vi "subReadIncrementalBuildInfoFromFile.vi"(8 "error in (no error)":errorcluster, 11 "SolutionBuilder in":refnum<class "SolutionBuilder.lvclass">) -> (0 "error out":errorcluster, 3 "SolutionBuilder out":refnum<class "SolutionBuilder.lvclass">)   [LabVIEW 2019, in "SolutionBuilder.lvlib" / "SolutionBuilder.lvclass"]
uses:
  SolutionBuilder.lvclass
  <vilib>/Utility/config.llb/NI_LVConfig.lvlib
  BuildManager/BuildProjectInfo.ctl
  BuildManager/BuildManager.lvclass
  IncrementalFileInfoHash.ctl
  <vilib>/Utility/miscctls.llb/LVMapReplaceAction.ctl
  <vilib>/Utility/config.llb/Read Key (String).vi
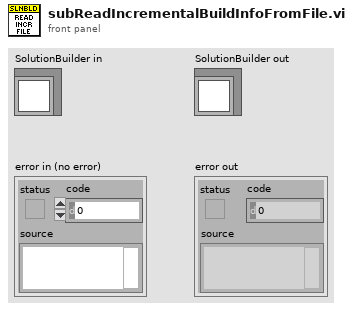
[diagram p1: front panel]
types:
  T1 = typedef "SolutionBuilder.lvlib/BuildManager.lvclass/BuildProjectInfo.ctl" = cluster{"Project path":string, "Build spec name":string, "Target":string}
  T2 = typedef "SolutionBuilder.lvlib/SolutionBuilder.lvclass/IncrementalFileInfoHash.ctl" = cluster{"Project path":string, "Build spec name":string, "Target":string, "File":string, "MD5 hash":string}
  T3 = typedef "LVMapReplaceAction.ctl" = enum32{"Modify Entry only if found", "Add or Modify Entry", "Delete Entry"}
  T4 = typedef "NI_LVConfig.lvlib/Config Data RefNum.ctl" = refnum<k1>
  T5 = typedef "SolutionBuilder.lvlib/SolutionBuilder.lvclass/HashMap.ctl" = map{T1, map{string, string}}
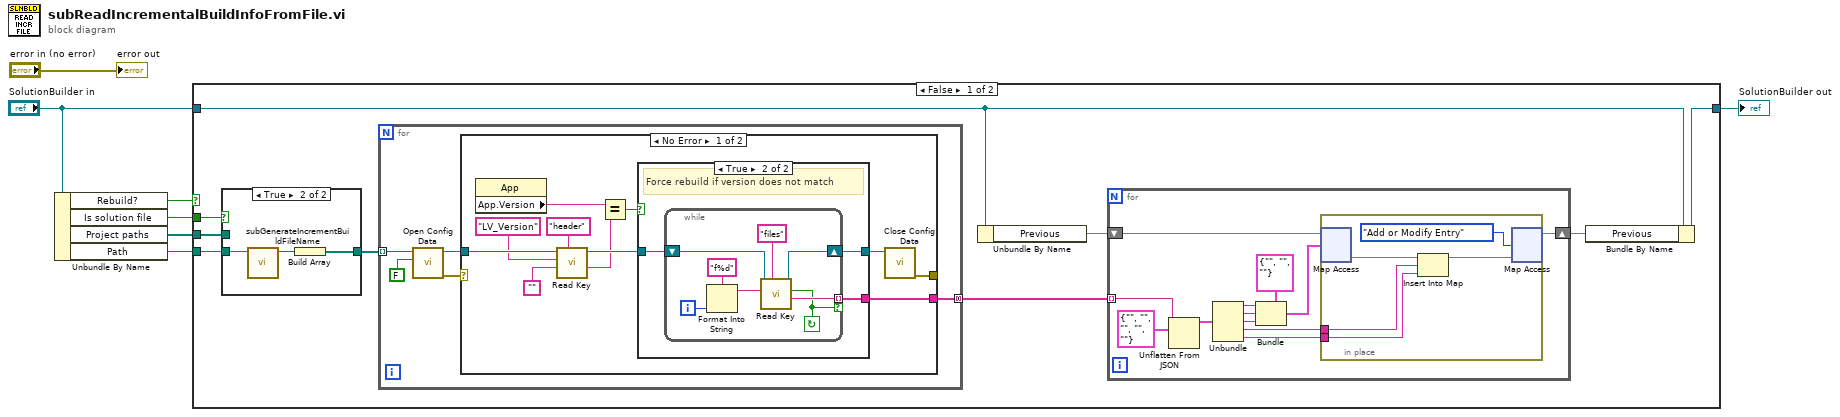
[diagram p0: block diagram]
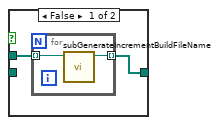
[diagram p4: hidden frame]
diagram:
  n1 = Unbundle By Name("SolutionBuilder in") -> ("Rebuild?"=w1:bool, "Is solution file"=w6:bool, "Project paths"=w4:path[], "Path"=w5:path)
  n2 = case shown="False" w1 {
    tunnel: w6 -> [w16 _]
    tunnel: w5 -> [w15 _]
    tunnel: w4 -> [w14 _]
    tunnel: [w10 w69] -> w3
    tunnel: "SolutionBuilder in" -> [w9 w69]
    frame False {
      n3 = case shown="True" w16 {
        tunnel: w15 -> [_ w51]
        tunnel: w14 -> [w46 _]
        tunnel: [w45 w49] -> w13
        frame False {
          n4 = for {
            tunnel: w46 -> [w48] mode=indexing
            tunnel: [w47] -> w45 mode=indexing
            n5 = call "subGenerateIncrementBuildFileName.vi"("Path in"=w48) -> ("Path out"=w47:path)  [unwired: 10 in]
          }
        }
        frame True {
          n6 = call "subGenerateIncrementBuildFileName.vi"("Path in"=w51) -> ("Path out"=w50:path)  [unwired: 10 in]
          n7 = Build Array(w50) -> (w49:path[])
        }
      }
      n8 = for {
        tunnel: w13 -> [w19] mode=indexing
        tunnel: [w18] -> w12 mode=concatenating
        n9 = call <vilib>:"Open Config Data.vi"("create file if necessary (T)"=FALSE, "configuration file path"=w19) -> ("error out"=w20:errorcluster, "refnum"=w21:T4)  [unwired: 7 in, 1 out]
        n10 = case shown="No Error" w20 {
          tunnel: w21 -> [w29 _]
          tunnel: [w31 _] -> _
          tunnel: [w30 _] -> w18
          frame No Error {
            n11 = property class="App"() -> ("App.Version"=w24:string)  [unwired: 2 in, 2 out]
            n12 = call-poly <vilib>:"Read Key.vi"("section"="header", "default value"="", "key"="LV_Version", "refnum"=w29) -> ("value"=w22:string, "refnum out"=w28:T4)  [unwired: 4 in, 2 out]
            n13 = Equal?(x=w24, y=w22) -> (x = y?=w23:bool)
            n14 = case shown="True" w23 {
              tunnel: [w33 w36] -> w32
              tunnel: [_ w35] -> w30
              tunnel: w28 -> [w33 w34]
              frame False {
              }
              frame True {
                # "Force rebuild if version does not match"
                n15 = while {
                  shift-right: [w40] -> w36
                  shift-left: w34 -> [w39]
                  tunnel: [w38] -> w35 mode=indexing if=w37
                  i -> [w41]
                  stop <- w37 continue-if-true
                  n16 = Format Into String(format string="f%d", w41) -> (resulting string=w43:string)  [unwired: 2 in, 1 out]
                  n17 = call-poly <vilib>:"Read Key.vi"("section"="files", "key"=w43, "refnum"=w39) -> ("value"=w38:string, "found?"=w37:bool, "refnum out"=w40:T4)  [unwired: 5 in, 1 out]
                }
              }
            }
            n18 = call <vilib>:"Close Config Data.vi"("refnum"=w32) -> ("error out"=w31:errorcluster)  [unwired: 9 in, 1 out]
          }
          frame Error {
          }
        }
      }
      n19 = Unbundle By Name(w9) -> ("Previous"=w8:T5)
      n20 = for {
        tunnel: w12 -> [w63] mode=indexing
        shift-right: [w55] -> w11
        shift-left: w8 -> [w57]
        n21 = Unflatten From JSON(JSON string=w63, type and defaults=T2 {"Project path"="", "Build spec name"="", "Target"="", "File"="", "MD5 hash"=""} ("cluster")) -> (value=w62:T2)  [unwired: 5 in, 1 out]
        n22 = Unbundle(w62) -> ("Project path"=w60:string, "Build spec name"=w59:string, "Target"=w54:string, "File"=w53:string, "MD5 hash"=w52:string)
        n23 = Bundle(cluster=T1 {"Project path"="", "Build spec name"="", "Target"=""}, "Project path"=w60, "Build spec name"=w59, "Target"=w54) -> (w56:T1)
        n24 = in-place {
          in-place-border: w53 -> [w66]
          in-place-border: w52 -> [w65]
          n25 = in-place-map #1(w57, w56) -> (w67:map{string, string})  [unwired: 1 in, 1 out]
          n26 = Insert Into Map(map in=w67, key=w66, value=w65) -> (map out=w64:map{string, string})  [unwired: 2 out]
          n27 = in-place-map #1(w64, LVMapReplaceAction."Add or Modify Entry" ("action")) -> (w55:T5)  [unwired: 2 out]
        }
      }
      n28 = Bundle By Name(cluster=w9, "Previous"=w11) -> (w10:refnum<class "SolutionBuilder.lvclass">)
    }
    frame True {
    }
  }
  "SolutionBuilder out" <- w3
  "error out" <- "error in (no error)"
